vi "Get Scaling Parameters (Table).vi"(0 "session in":refnum<k21>, 5 "physical channel":refnum<k21>="$DefaultPhysChans", 11 "error in (no error)":errorcluster) -> (4 "session out":refnum<k21>, 6 "physical channel out":refnum<k21>, 8 "scaled values":dbl[](array[numeric]), 10 "pre-scaled values":dbl[](array[numeric]), 14 "coercion":i32(ring) items=["Interpolate", "RoundToNearest", "Strict"], 15 "error out":errorcluster)   [LabVIEW 2020, in "SLSC.lvlib"]
doc: "Gets scaling parameters from a table scale that maps an array of pre-scaled values to an array of corresponding scaled values."
uses:
  <vilib>/SLSC/SLSC.lvlib
  nislsclvapi.dll
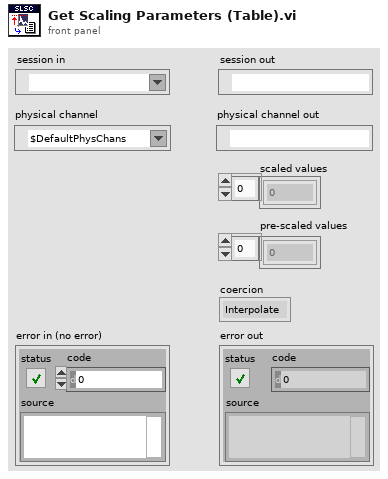
[diagram p1: front panel]
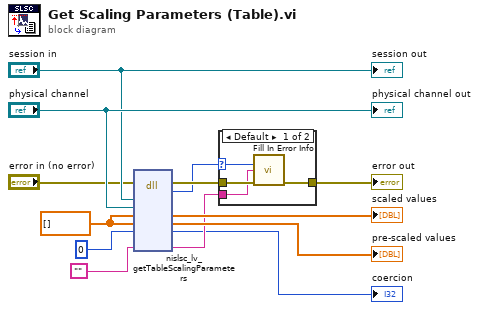
[diagram p0: block diagram]
diagram:
  w9 = dbl[] [] ("scaledValues")
  n1 = dll-call lib="nislsclvapi.*" fn="nislsc_lv_getTableScalingParameters"(error in="error in (no error)", "session"="session in", "physical channel"="physical channel", "scaledValues"=w9, "prescaleValues"=w9, "coercion"=0, "extendedErrorInfo"="") -> (error out=w6:errorcluster, "return type"=w3:i32, "scaledValues"=→"scaled values":dbl[], "prescaleValues"=→"pre-scaled values":dbl[], "coercion"=→"coercion":i32, "extendedErrorInfo"=w4:string)  [unwired: 6 in, 1 out]
  n2 = case shown="Default" w3 {
    selector: w3 -> [w14 _]
    tunnel: w4 -> [w15 _]
    tunnel: w6 -> [w17 w18]
    tunnel: [w16 w18] -> w5
    frame Default {
      n3 = call <vilib>:"Fill In Error Info.vi"("status code"=w14, "extended error info"=w15, "error in"=w17) -> ("error out"=w16:errorcluster)  [unwired: 12 in]
    }
    frame 0 {
    }
  }
  "error out" <- w5
  "session out" <- "session in"
  "physical channel out" <- "physical channel"
